vi "SaveExperimentInfo.vi"(10 "File path":path=path "D:/labview/jelmer/labview tmp/measureinfo.txt", 11 "MeasureConfig":T13={"Bead locations"=[{"X"=0, "Y"=0}], "ROI"=0, "Experiment base path"=path "", "Image output subdir"="images", "Output mode"=enum."None", "Traces output subdir"="traces", "QTrk Settings"={"Image width"=150, "Image height"=150, "Number of threads (CPU based)"=-1, "CUDA Device"=200, "COM Background correction factor"=128.0, "ZLUT MinRadius"=32.0, "ZLUT Radial sample density"=2.0, "ZLUT Angular sample density"=5.0, "ZLUT ROI Coverage"=50.0, "QI Iterations"=64, "QI MinRadius"=2.0, "QI Radial sample density"=64.0, "QI Angular sample density"=64.0, "QI ROI Coverage"=2.0, "QI Angular Step \nIteration Factor"=30.0, "XCOR Profile Length"=0, "XCOR Profile Width"=2, "XCOR Iterations"=32, "Gaussian 2D Fit Iterations"=8, "Gaussian 2D Sigma (pixels)"=3.0, "Downsample"=0}, "Tracking Config"={"Number of steps"=150, "ZLUT stepsize (um)"=150.0, "Z correction factor"=-1.0, "Start piezo Z (um)"=200.0, "Pixel size (nm)"=128.0, "2D Localization Type"=enum."Quadrant Interpolation", "Z Command (None)"=enum."Nothing", "Z Piezo scale"=FALSE}, "Experiment Name"="", "Program"={"Commands"=[], "Motor Axis accuracy conditions"={"Magnet Z"=0.0, "Magnet rotation"=0.0, "Camera"={"X"=0.0, "Y"=0.0}, "Piezo XY"={"X"=0.0, "Y"=0.0}, "Piezo Z"=0.0}, "Axis flags"={"Magnet Z"=FALSE, "Magnet rotation"=FALSE, "Camera"={"X"=FALSE, "Y"=FALSE}, "Piezo XY"={"X"=FALSE, "Y"=FALSE}, "Piezo Z"=FALSE}}, "ZLUT"=[], "Camera settings"={"Framerate (Hz)"=60, "Exposure time (us)"=5000, "Image size"={"Width"=1280, "Height"=1024}, "Number of buffers"=30}, "Experiment Script"="", "Max frames in memory"=2, "Save traces as binary"=FALSE, "Pixel Calibration Gain Image"="camera_calib_gain.bin", "Pixel Calibration Offset Image"="camera_calib_gain.bin", "Use pixel calibration images"=FALSE, "Internal camera settings"="", "Trace write interval"=100} {"QTrk Settings"."QI ROI Coverage" format="%_2g"; "QTrk Settings"."QI MinRadius" format="%.2f"; "QTrk Settings"."QI Angular sample density" format="%.3f"; "QTrk Settings"."QI Radial sample density" format="%.2f"; "QTrk Settings"."ZLUT Radial sample density" format="%.2f"; "QTrk Settings"."ZLUT MinRadius" format="%.2f"}) -> ()   [LabVIEW 2011]
uses:
  Typedefs/MeasureConfigType.ctl
  Typedefs/MeasureConfigOutputMode.ctl
  qtrk/QTrkLVBinding/QTrkSettings.ctl
  Typedefs/TrackingConfigType.ctl
  qtrk/QTrkLVBinding/QTrkLocalizationType.ctl
  qtrk/QTrkLVBinding/QTrkZCommandType.ctl
  ExperimentProgram/ExperimentProgramType.ctl
  ExperimentProgram/ExProgCommandType.ctl
  ExperimentProgram/ExProgCommandEnumType.ctl
  Motors/MotorAxisEnum.ctl
  Motors/MotorPosType.ctl
  Typedefs/XYf.ctl
  Motors/MotorPosFlagsType.ctl
  Camera/GenericCameraConfigType.ctl
panel:
  out "data to save":T12={"ROI"=0, "Experiment base path"=path "", "QTrk Settings"={"Image width"=0, "Image height"=0, "Number of threads (CPU based)"=0, "CUDA Device"=0, "COM Background correction factor"=0.0, "ZLUT MinRadius"=0.0, "ZLUT Radial sample density"=0.0, "ZLUT Angular sample density"=0.0, "ZLUT ROI Coverage"=0.0, "QI Iterations"=0, "QI MinRadius"=0.0, "QI Radial sample density"=0.0, "QI Angular sample density"=0.0, "QI ROI Coverage"=0.0, "QI Angular Step \nIteration Factor"=0.0, "XCOR Profile Length"=0, "XCOR Profile Width"=0, "XCOR Iterations"=0, "Gaussian 2D Fit Iterations"=0, "Gaussian 2D Sigma (pixels)"=3.0, "Downsample"=0}, "Tracking Config"={"Number of steps"=0, "ZLUT stepsize (um)"=0.0, "Z correction factor"=0.0, "Start piezo Z (um)"=0.0, "Pixel size (nm)"=0.0, "2D Localization Type"=enum."Quadrant Interpolation", "Z Command (None)"=enum."Nothing", "Z Piezo scale"=FALSE}, "Image output subdir"="", "Traces output subdir"="", "Output mode"=enum."None", "Camera settings"=variant, "Experiment Name"="", "Program"={"Commands"=[], "Motor Axis accuracy conditions"={"Magnet Z"=0.0, "Magnet rotation"=0.0, "Camera"={"X"=0.0, "Y"=0.0}, "Piezo XY"={"X"=0.0, "Y"=0.0}, "Piezo Z"=0.0}, "Axis flags"={"Magnet Z"=FALSE, "Magnet rotation"=FALSE, "Camera"={"X"=FALSE, "Y"=FALSE}, "Piezo XY"={"X"=FALSE, "Y"=FALSE}, "Piezo Z"=FALSE}}}
  out "ValueList (out)":cluster{"Label":string, "Variant":variant}[](array[cluster])
  # "-2: Use all devices\n-1: Use best device"
  # "(used for commands with string parameters)"
  # "(used for commands with string parameters)"
  # "-2: Use all devices\n-1: Use best device"
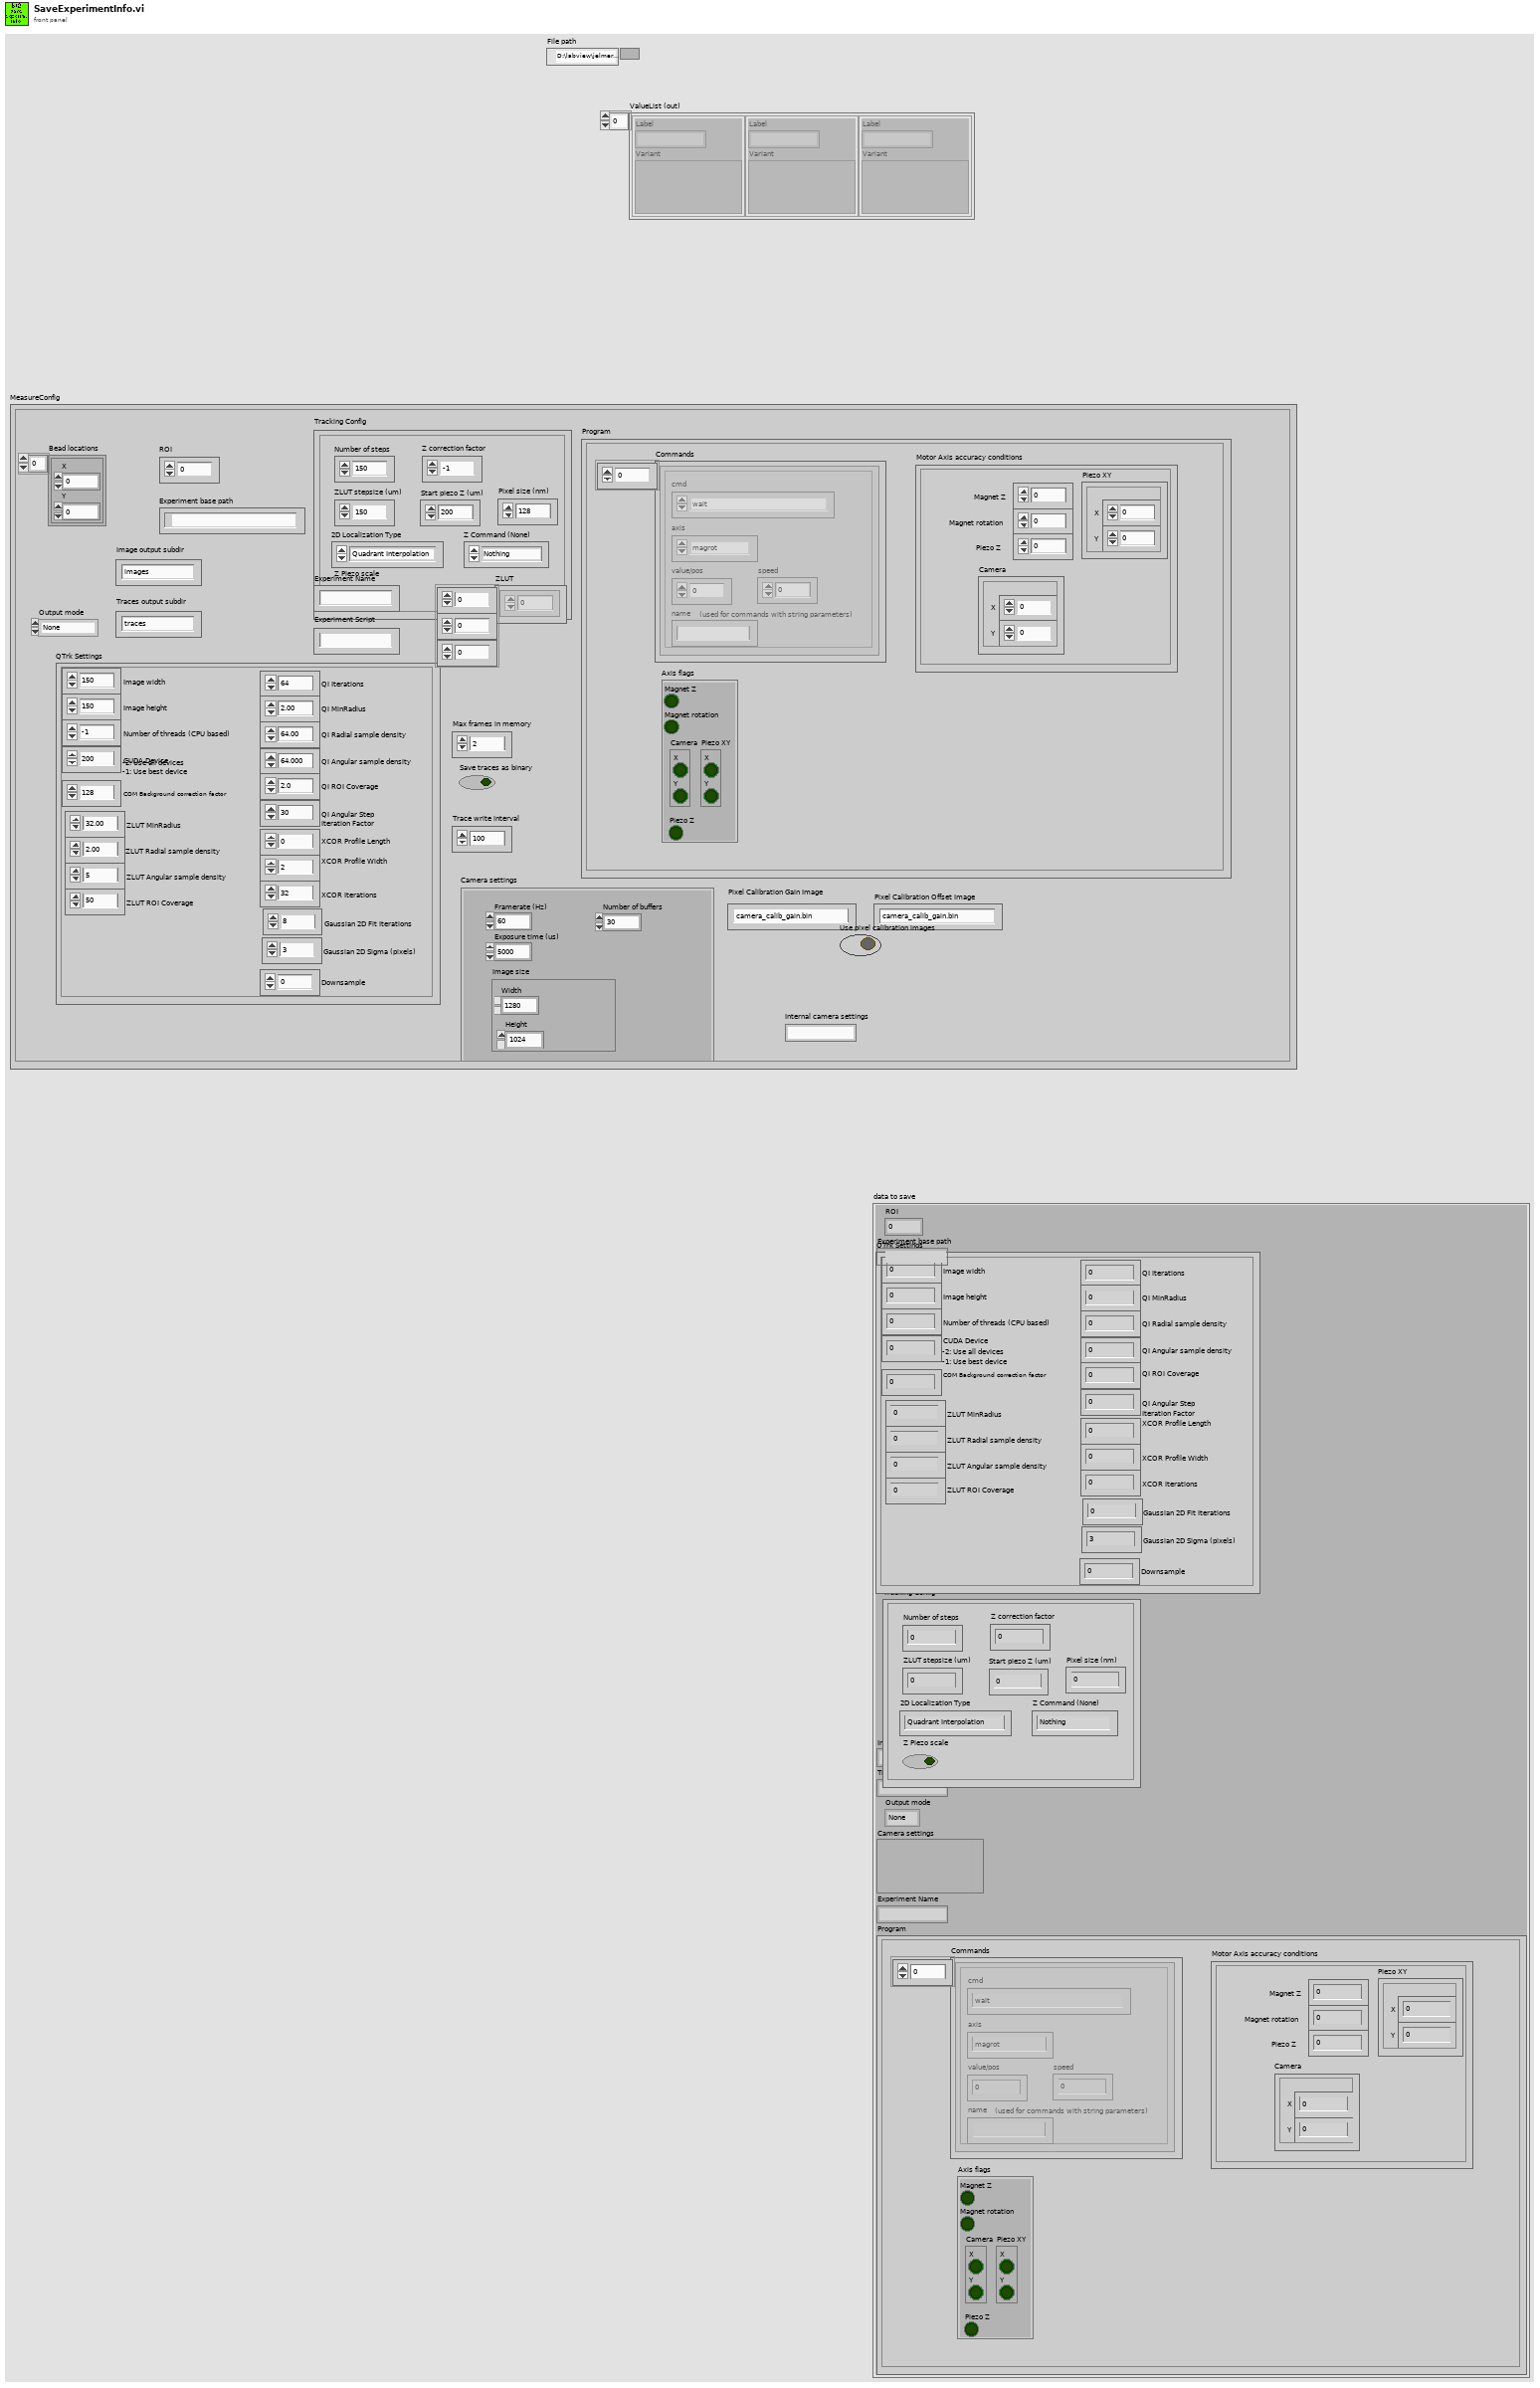
[diagram p1: front panel]
types:
  T1 = typedef "QTrkSettings.ctl" = cluster{"Image width":i32, "Image height":i32, "Number of threads (CPU based)":i32, "CUDA Device":i32, "COM Background correction factor":sgl, "ZLUT MinRadius":sgl, "ZLUT Radial sample density":sgl, "ZLUT Angular sample density":sgl, "ZLUT ROI Coverage":sgl, "QI Iterations":i32, "QI MinRadius":sgl, "QI Radial sample density":sgl, "QI Angular sample density":sgl, "QI ROI Coverage":sgl, "QI Angular Step \nIteration Factor":sgl, "XCOR Profile Length":i32, "XCOR Profile Width":i32, "XCOR Iterations":i32, "Gaussian 2D Fit Iterations":i32, "Gaussian 2D Sigma (pixels)":sgl, "Downsample":i32}
  T2 = typedef "TrackingConfigType.ctl" = cluster{"Number of steps":i32, "ZLUT stepsize (um)":sgl, "Z correction factor":sgl, "Start piezo Z (um)":sgl, "Pixel size (nm)":sgl, "2D Localization Type":T3, "Z Command (None)":T4, "Z Piezo scale":bool}
  T3 = typedef "QTrkLocalizationType.ctl" = enum16{"Center-of-Mass", "1D Cross-Correlation", "Quadrant Interpolation", "Gaussian 2D MLE", "QI + ZLUTAlign", "ZLUTAlign", "QI + FourierLUT"}
  T4 = typedef "QTrkZCommandType.ctl" = enum16{"Nothing", "ComputeZ", "BuildRadialZLUT", "BuildImageZLUT", "RadialZLUT+ImageZLUT"}
  T5 = typedef "ExperimentProgramType.ctl" = cluster{"Commands":T6[], "Motor Axis accuracy conditions":T9, "Axis flags":T11}
  T6 = typedef "ExProgCommandType.ctl" = cluster{"cmd":T7, "axis":T8, "value/pos":dbl, "speed":dbl, "name":string}
  T7 = typedef "ExProgCommandEnumType.ctl" = enum16{"wait", "move", "acquire", "idle", "rmove", "when", "section", "stop"}
  T8 = typedef "MotorAxisEnum.ctl" = enum16{"no axis", "magrot", "magpos", "px", "py", "pz", "camx", "camy"}
  T9 = typedef "MotorPosType.ctl" = cluster{"Magnet Z":dbl, "Magnet rotation":dbl, "Camera":T10, "Piezo XY":T10, "Piezo Z":dbl}
  T10 = typedef "XYf.ctl" = cluster{"X":sgl, "Y":sgl}
  T11 = typedef "MotorPosFlagsType.ctl" = cluster{"Magnet Z":bool, "Magnet rotation":bool, "Camera":cluster{"X":bool, "Y":bool}, "Piezo XY":cluster{"X":bool, "Y":bool}, "Piezo Z":bool}
  T12 = cluster{"ROI":i32, "Experiment base path":path, "QTrk Settings":T1, "Tracking Config":T2, "Image output subdir":string, "Traces output subdir":string, "Output mode":enum16{"None", "Track", "SaveImages"}, "Camera settings":variant, "Experiment Name":string, "Program":T5}
  T13 = typedef "MeasureConfigType.ctl" = cluster{"Bead locations":cluster{"X":i32, "Y":i32}[], "ROI":i32, "Experiment base path":path, "Image output subdir":string, "Output mode":T14, "Traces output subdir":string, "QTrk Settings":T1, "Tracking Config":T2, "Experiment Name":string, "Program":T5, "ZLUT":sgl[][][], "Camera settings":T15, "Experiment Script":string, "Max frames in memory":i32, "Save traces as binary":bool, "Pixel Calibration Gain Image":string, "Pixel Calibration Offset Image":string, "Use pixel calibration images":bool, "Internal camera settings":string, "Trace write interval":i32}
  T14 = typedef "MeasureConfigOutputMode.ctl" = enum16{"None", "Track", "SaveImages"}
  T15 = typedef "GenericCameraConfigType.ctl" = cluster{"Framerate (Hz)":i32, "Exposure time (us)":i32, "Image size":cluster{"Width":i32, "Height":i32}, "Number of buffers":i32}
  T16 = cluster{"ROI":i32, "Experiment base path":path, "QTrk Settings":T1, "Tracking Config":T2, "Image output subdir":string, "Traces output subdir":string, "Output mode":T14, "Camera settings":T15, "Experiment Name":string, "Program":T5}
  T17 = enum16{"None", "Normalize", "NormalizeWithoutOffset"}
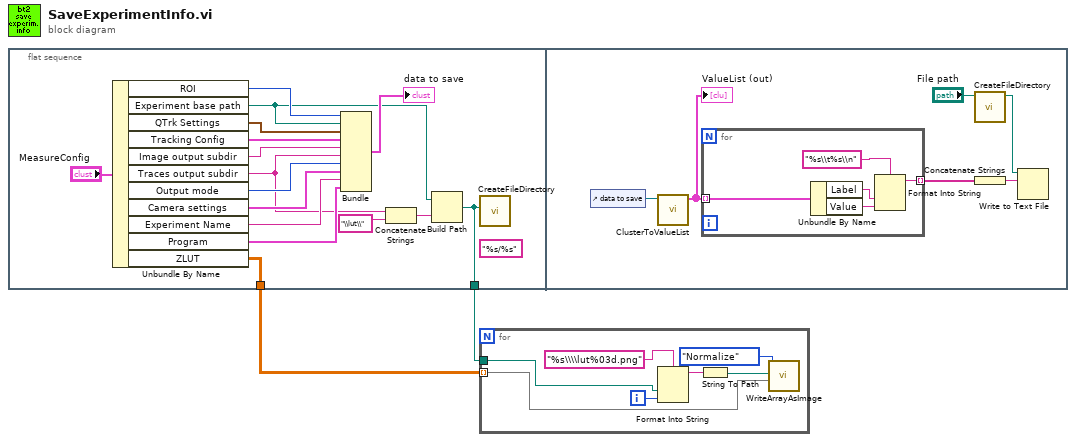
[diagram p0: block diagram]
diagram:
  n1 = flat-sequence {
    tunnel: [w6] -> w2
    tunnel: [w8] -> w1
    frame #0 {
      (unwired) "%s/%s" ("format string")
      n2 = Unbundle By Name("MeasureConfig") -> ("ROI"=w18:i32, "Experiment base path"=w7:path, "QTrk Settings"=w17:T1, "Tracking Config"=w16:T2, "Image output subdir"=w15:string, "Traces output subdir"=w5:string, "Output mode"=w14:T14, "Camera settings"=w13:T15, "Experiment Name"=w12:string, "Program"=w11:T5, "ZLUT"=w8:sgl[][][])
      n3 = Bundle("ROI"=w18, "Experiment base path"=w7, "QTrk Settings"=w17, "Tracking Config"=w16, "Image output subdir"=w15, "Traces output subdir"=w5, "Output mode"=w14, "Camera settings"=w13, "Experiment Name"=w12, "Program"=w11) -> (→"data to save":T16)  [unwired: 1 in]
      n4 = Concatenate Strings(w5, "\\lut\\" ("string")) -> (w3:string)
      n5 = Build Path(base path=w7, name or relative path=w3) -> (appended path=w6:path)
      n6 = call "CreateFileDirectory.vi"("directory"=w6) -> ()  [unwired: 10 in, 1 out]
    }
    frame #1 {
      n7 = control-ref of="data to save"() -> (w19:refnum<vi>)
      n8 = call "ClusterToValueList.vi"("Cluster Refnum"=w19) -> ("ValueList (out)"=w23:cluster{"Label":string, "Value":string}[])  [unwired: 10 in]
      "ValueList (out)" <- w23
      n9 = for {
        tunnel: w23 -> [w27] mode=indexing
        tunnel: [w26] -> w22 mode=indexing
        n10 = Unbundle By Name(w27) -> ("Label"=w29:string, "Value"=w25:string)
        n11 = Format Into String(format string="%s\\t%s\\n", w29, w25) -> (resulting string=w26:string)  [unwired: 2 in, 1 out]
      }
      n12 = call "CreateFileDirectory.vi"("filename"="File path") -> ("filename (copy)"=w20:path)  [unwired: 10 in]
      n13 = Concatenate Strings(w22) -> (w24:string)
      n14 = Write to Text File(file (use dialog)=w20, text=w24) -> ()  [unwired: 2 in, 3 out]
    }
  }
  n15 = for {
    tunnel: w2 -> [w35]
    tunnel: w1 -> [w36] mode=indexing
    i -> [w31]
    n16 = Format Into String(format string="%s\\\\lut%03d.png", w35, w31) -> (resulting string=w33:string)  [unwired: 2 in, 1 out]
    n17 = String To Path(string=w33) -> (path=w32:path)
    n18 = call "WriteArrayAsImage.vi"("Data"=w36, "File Path"=w32, "Normalize Mode"=T17."Normalize") -> ()  [unwired: 9 in]
  }
